vi "Square Root 03.vi"(1 "x":sgl) -> (0 "sqrt(x)":sgl)   [LabVIEW 2015]
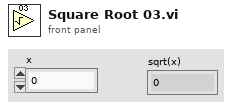
[diagram p1: front panel]
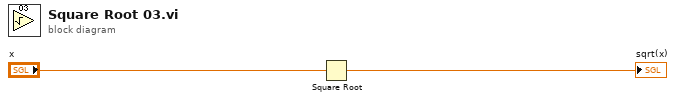
[diagram p0: block diagram]
diagram:
  n1 = Square Root(x="x") -> (sqrt(x)=→"sqrt(x)":sgl)
